vi "Signal_Scale.vi"() -> ()   [LabVIEW 2018]
panel:
  in  "stop":bool
  in  "Амплитуда":dbl(knob) scale=0.0..10.0
  out "Waveform Chart":dbl(graph)
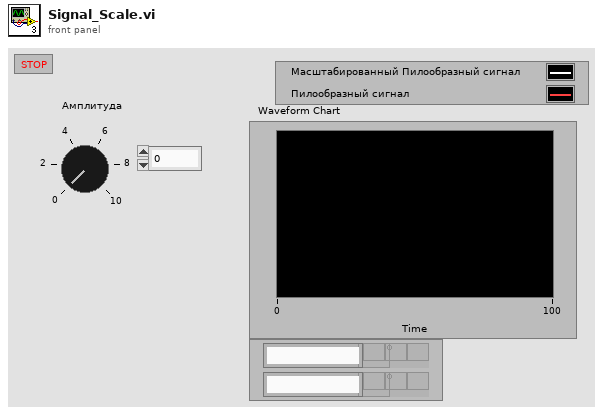
[diagram p1: front panel]
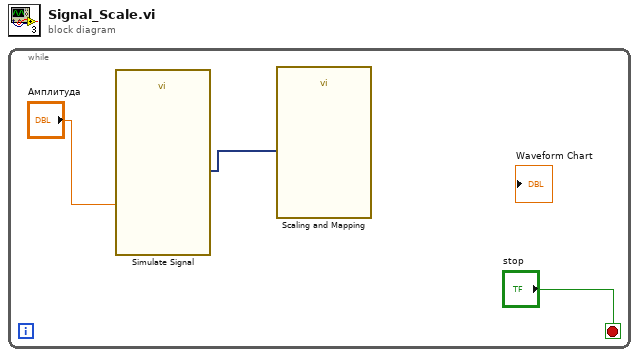
[diagram p0: block diagram]
diagram:
  n1 = while {
    stop <- "stop" stop-if-true
    n2 = call "Simulate Signal"("Amplitude"="Амплитуда") -> ("Sawtooth"=w1:dynamicdata)  [unwired: 13 in, 1 out]
    n3 = call "Scaling and Mapping"("Signals"=w1) -> ()  [unwired: 9 in, 2 out]
  }
